vi "TimedLog.vi"(8 "error in (no error)":errorcluster, 10 "Message":string, 11 "Logger in":refnum<class "Logger.lvclass">) -> (0 "error out":errorcluster, 2 "logged string":string, 3 "Logger out":refnum<class "Logger.lvclass">)   [LabVIEW 2011, in "Logger.lvclass"]
doc: "Concatenates the current time to the beginning of the provided \"Message\" before it is sent to the Log method. The Logger Object will write this time-stamped message to a log (text) file by a background process.\n\nJared Kirschner, 2012."
uses:
  Logger.lvclass
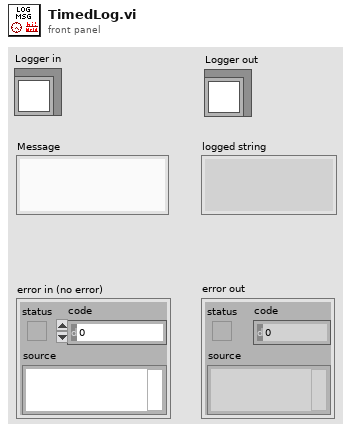
[diagram p1: front panel]
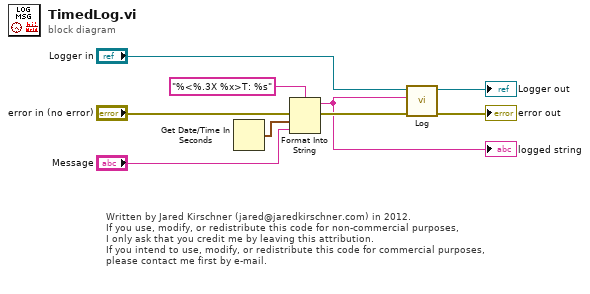
[diagram p0: block diagram]
diagram:
  # "Written by Jared Kirschner (jared@jaredkirschner.com) in 2012.\nIf you use, modify, or redistribute this code for non-commercial purposes,\nI only ask that you credit me by leaving this attribution.\nIf you intend to use, modify, or redistribute this code for commercial purposes,\nplease contact me first by e-mail."
  n1 = Get Date/Time In Seconds() -> (seconds since 1Jan1904=w5:timestamp)
  n2 = Format Into String(format string="%<%.3X %x>T: %s" ("initial string"), error in="error in (no error)", w5, "Message") -> (resulting string=w6:string, error out=w7:errorcluster)  [unwired: 1 in]
  "logged string" <- w6
  n3 = call "Log.vi"("error in (no error)"=w7, "Message"=w6, "Logger in"="Logger in") -> ("error out"=→"error out":errorcluster, "Logger out"=→"Logger out":refnum<class "Logger.lvclass">)  [unwired: 7 in]
